vi "Write IQ_to_VQ.vi"(8 "error in (no error)":errorcluster, 10 "PI_Settings":T1={"gains"={"proportional gain"=0.0, "integral gain"=0.0}, "output range"={"output high (Inf)"=inf, "output low (-Inf)"=-inf}, "PI_state"=enum."idle", "reset"=FALSE, "manual"=0.0} {"gains"."proportional gain" step=0.125}, 11 "ActiveFrontEndModule configuration in":refnum<class "ActiveFrontEndModule configuration.lvclass">) -> (0 "error out":errorcluster, 3 "ActiveFrontEndModule configuration out":refnum<class "ActiveFrontEndModule configuration.lvclass">)   [LabVIEW 2017, in "ActiveFrontEndModule configuration.lvclass"]
uses:
  ActiveFrontEndModule configuration.lvclass
  <vilib>/NI/PowerElectronicsControl/ActiveFrontEnd/AFE/PI_Settings.ctl
  <vilib>/rvi/Analysis/control/PID/Typedef/niFpgaPID_PIGains.ctl
  <vilib>/rvi/Analysis/control/PID/Typedef/niFpgaPID_OutputRange.ctl
  ActiveFrontEndModule configuration.lvclass/ActiveFrontEndModule configuration.ctl
  <vilib>/NI/PowerElectronicsControl/ActiveFrontEnd/AFE/ActiveFrontEnd.lvlib
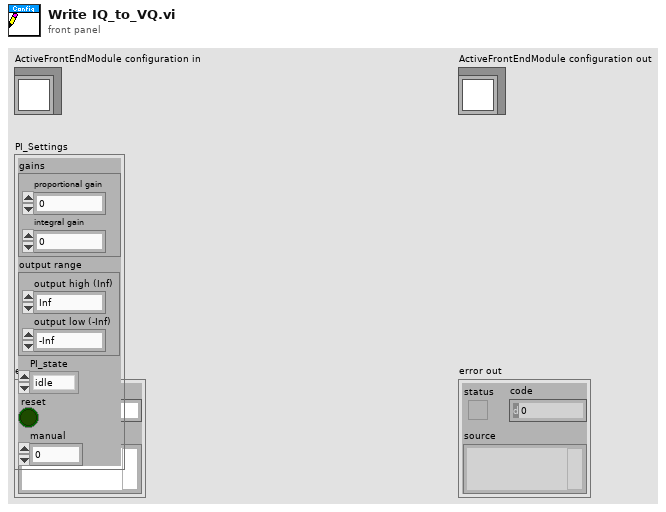
[diagram p1: front panel]
types:
  T1 = typedef "ActiveFrontEnd.lvlib/PI_Settings.ctl" = cluster{"gains":T2, "output range":T3, "PI_state":enum8{"idle", "normal", "manual", "perturbance"}, "reset":bool, "manual":sgl}
  T2 = typedef "niFpgaPID_PIGains.ctl" = cluster{"proportional gain":sgl, "integral gain":sgl}
  T3 = typedef "niFpgaPID_OutputRange.ctl" = cluster{"output high (Inf)":sgl, "output low (-Inf)":sgl}
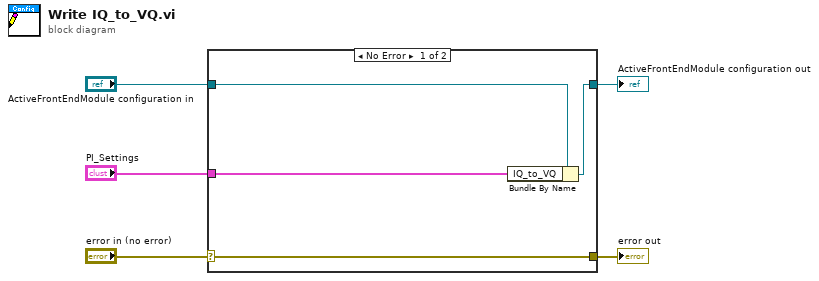
[diagram p0: block diagram]
diagram:
  n1 = case shown="No Error" "error in (no error)" {
    selector: "error in (no error)" -> [w9 w10]
    tunnel: [w9 w10] -> w4
    tunnel: [w7 w11] -> w2
    tunnel: "ActiveFrontEndModule configuration in" -> [w8 w11]
    tunnel: "PI_Settings" -> [w6 _]
    frame No Error {
      n2 = Bundle By Name(cluster=w8, "IQ_to_VQ"=w6) -> (w7:refnum<class "ActiveFrontEndModule configuration.lvclass">)
    }
    frame Error {
    }
  }
  "error out" <- w4
  "ActiveFrontEndModule configuration out" <- w2
